vi "ModHeaderFilePar.vi"() -> ()   [LabVIEW 2019]
uses:
  Interface Class/ScanParams.ctl
  Interface Class/ScanParamsOld.ctl
  Interface Class/Interface.lvclass
panel:
  out "Header Scan":i64[](array[numeric])
  out "Session#":bool[](array[boolean])
  out "scan#":bool[](array[boolean])
  out "ScanParamsOut":T1[](array[typedef])
  out "ScanPar":i32[](array[numeric])
  out "ChainePar":string[](array[string])
  out "Session":i32[](array[numeric])
  out "Tableau 2":i32[](array[numeric])
  out "Reste session":string[](array[string])
  out "offset scan":i32[](array[numeric])
  out "ChaineSession":string[](array[string])
  out "Scan":i32[](array[numeric])
  out "Années":i32[](array[numeric])
  out "Tous Mois":i32[](array[numeric])
  out "Jours":i32[](array[numeric])
  out "ChaineReste":string[](array[string])
  out "Tableau":string[](array[string])
  out "HdrFilesNames":path[](array[path])
  in  "Data Folder Path":path
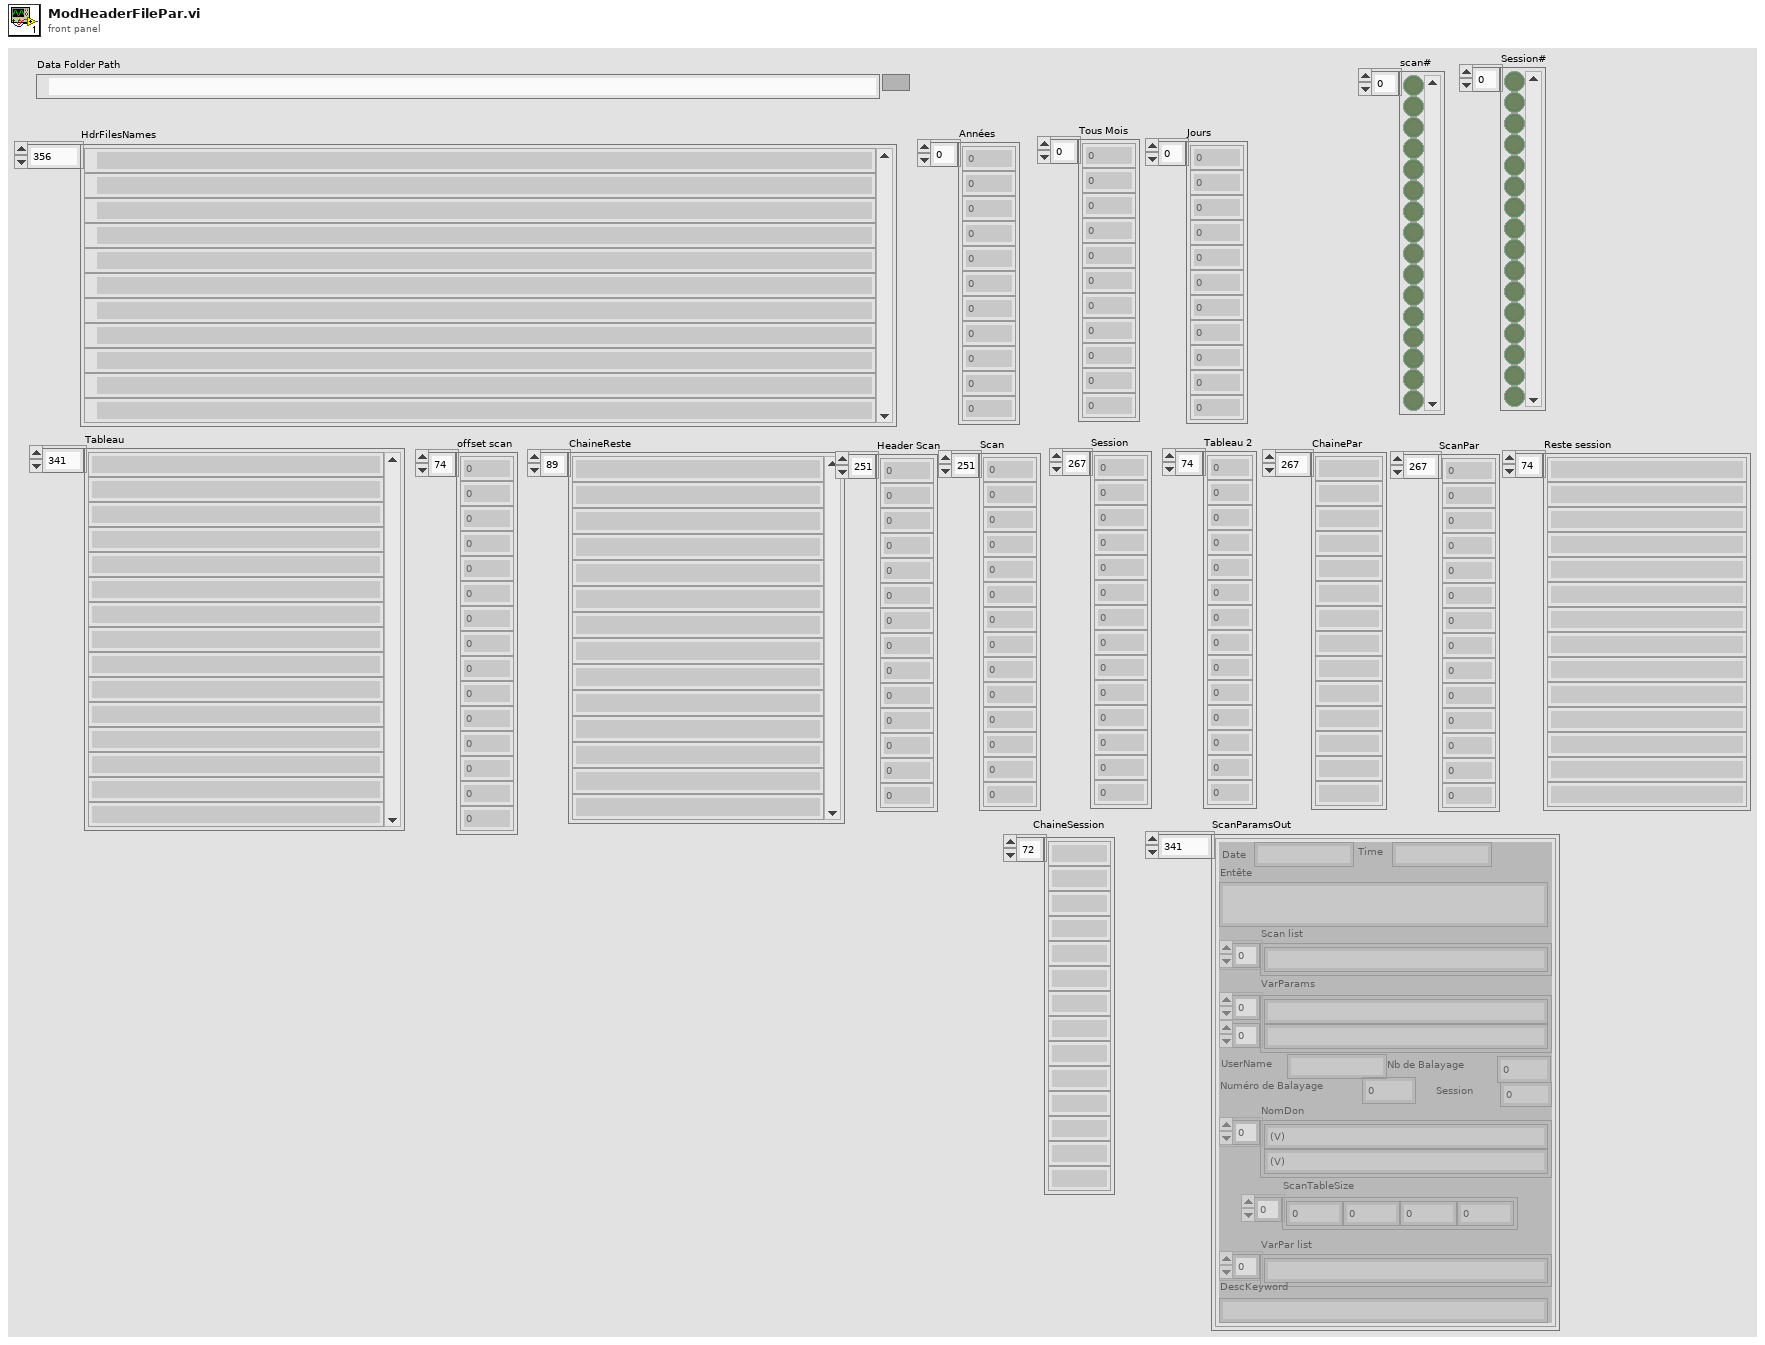
[diagram p1: front panel]
types:
  T1 = typedef "Interface.lvclass/ScanParams.ctl" = cluster{"Entête":string, "Scan list":string[], "NbCourbe":i32, "IndCourbe":i64, "NomDon":string[], "Session ":i32, "Date":string, "Time":string, "VarParams":string[][], "UserName":string, "ScanTableSize":i32[], "VarPar list":string[], "DescKeyword":string}
  T2 = typedef "Interface.lvclass/ScanParamsOld.ctl" = cluster{"Entête":string, "Scan list":string[], "NbCourbe":i32, "IndCourbe":i64, "NomDon":string[], "Session ":i32, "Date":string, "Time":string, "VarParams":string[][], "UserName":string, "ScanTableSize":i32[], "VarPar list":string[]}
  T3 = enum16{"open", "replace", "create", "open or create", "replace or create", "replace or create with confirmation"}
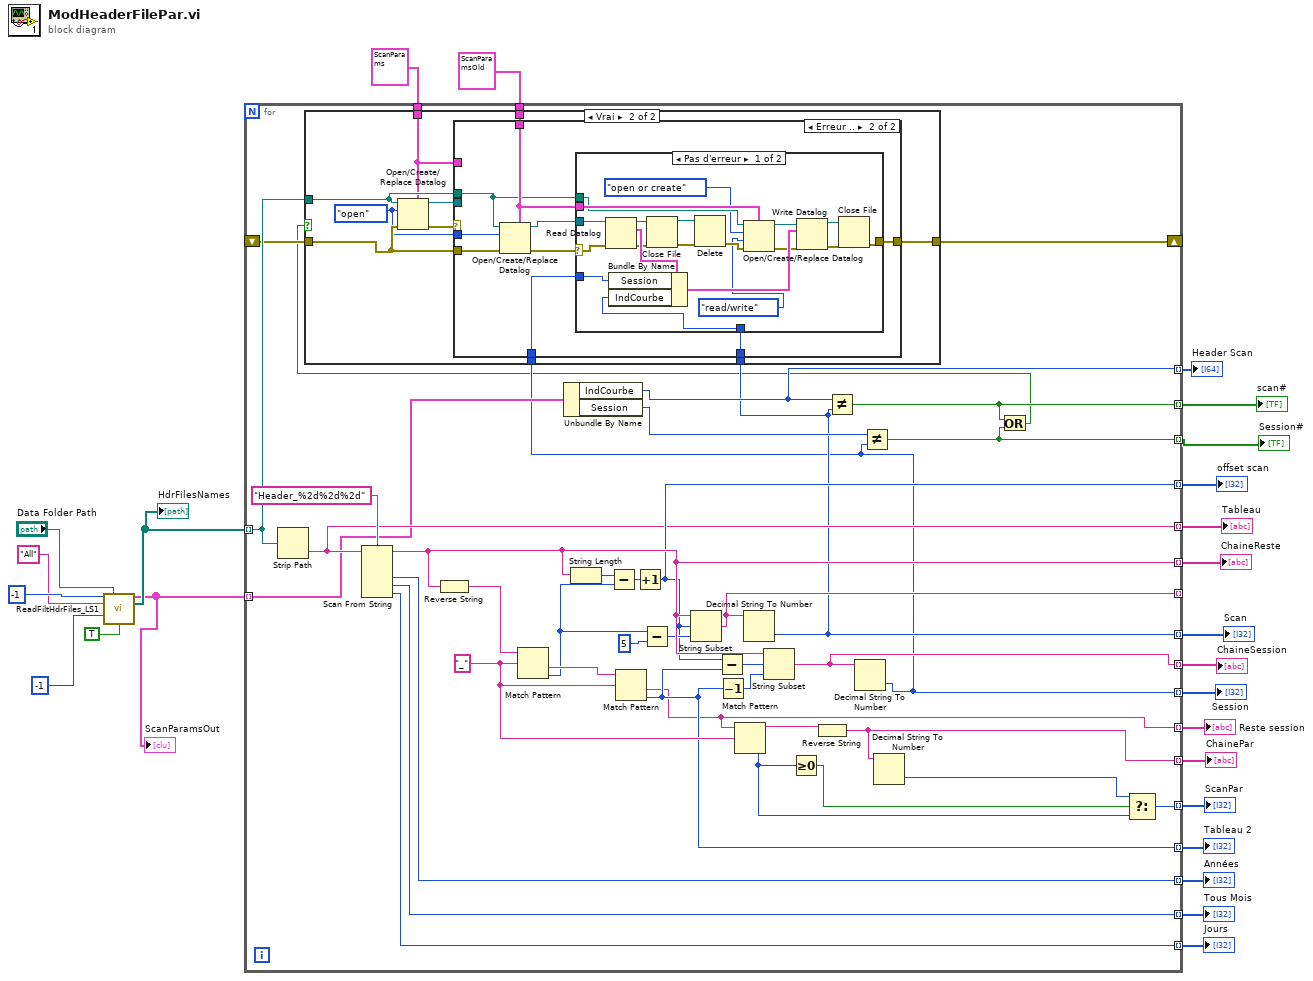
[diagram p0: block diagram]
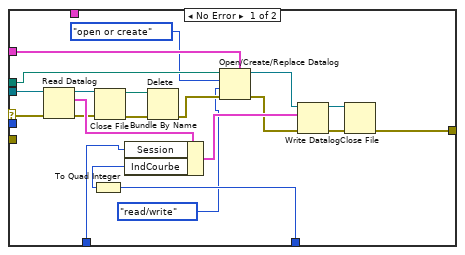
[diagram p3: hidden frame]
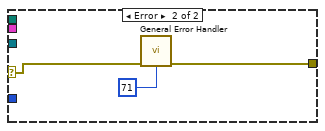
[diagram p4: hidden frame]
diagram:
  n1 = call "ReadFiltHdrFiles_LS1.vi"("nombre (-1)"=-1, "Data Folder Path"="Data Folder Path", "Date String"="All", "Session"=-1, "Recheck Files"=TRUE) -> ("ScanParamsOut"=w6:T1[], "FilesPath"=w7:path[])  [unwired: 8 in, 1 out]
  "HdrFilesNames" <- w7
  "ScanParamsOut" <- w6
  n2 = for {
    tunnel: w7 -> [w35] mode=indexing
    tunnel: [w47] -> w25 mode=indexing
    tunnel: [w58] -> w24 mode=indexing
    tunnel: [w64] -> w23 mode=indexing
    tunnel: [w63] -> w22 mode=indexing
    tunnel: [w62] -> w21 mode=indexing
    tunnel: [w30] -> w20 mode=indexing
    tunnel: [w46] -> w19 mode=indexing
    tunnel: [w56] -> _ mode=indexing
    tunnel: [w52] -> w18 mode=indexing
    tunnel: [w45] -> w17 mode=indexing
    tunnel: [w48] -> w16 mode=indexing
    tunnel: [w29] -> w15 mode=indexing
    tunnel: [w39] -> w14 mode=indexing
    tunnel: [w41] -> w13 mode=indexing
    tunnel: w6 -> [w38] mode=indexing
    tunnel: [w28] -> w5 mode=indexing
    tunnel: [w27] -> w4 mode=indexing
    tunnel: [w36] -> w3 mode=indexing
    shift-right: [w32] -> _
    shift-left: _ -> [w33]
    tunnel: T1 {"Entête"="", "Scan list"=[], "NbCourbe"=1, "IndCourbe"=1, "NomDon"=["RTêta;", "X&Y;"], "Session "=0, "Date"="", "Time"="", "VarParams"=[], "UserName"="", "ScanTableSize"=[], "VarPar list"=[], "DescKeyword"=""} ("ScanParams") -> [w34]
    tunnel: T2 {"Entête"="", "Scan list"=[], "NbCourbe"=1, "IndCourbe"=0, "NomDon"=["RTêta;", "X&Y;"], "Session "=0, "Date"="", "Time"="", "VarParams"=[], "UserName"="", "ScanTableSize"=[], "VarPar list"=[]} ("ScanParams") -> [w31]
    w60 = "_" ("expression régulière")
    n3 = Strip Path(path=w35) -> (name=w47:string)  [unwired: 1 out]
    n4 = Scan From String(format string="Header_%2d%2d%2d" ("chaîne de format"), input string=w47) -> (remaining string=w58:string, output 1=w62:i32, output 2=w63:i32, output 3=w64:i32)  [unwired: 5 in, 2 out]
    n5 = Reverse String(1:w58) -> (0:w61:string)
    n6 = Match Pattern(string=w61, regular expression=w60) -> (after substring=w51:string, offset past match=w50:i32)  [unwired: 1 in, 2 out]
    n7 = Unbundle By Name(w38) -> ("IndCourbe"=w36:i64, "Session"=w37:i32)
    n8 = String Length(string=w58) -> (length=w59:i32)
    n9 = Subtract(x=w59, y=w50) -> (x-y=w55:i32)
    n10 = Match Pattern(string=w51, regular expression=w60) -> (after substring=w45:string, offset past match=w48:i32)  [unwired: 1 in, 2 out]
    n11 = Increment(x=w55) -> (x+1=w52:i32)
    n12 = Subtract(x=w50, y=5) -> (x-y=w54:i32)
    n13 = String Subset(string=w58, offset (0)=w52, length (rest)=w54) -> (substring=w56:string)
    n14 = Subtract(x=w52, y=w48) -> (x-y=w57:i32)
    n15 = Decrement(x=w48) -> (x-1=w49:i32)
    n16 = Match Pattern(string=w45, regular expression=w60) -> (before substring=w40:string, offset past match=w42:i32)  [unwired: 1 in, 2 out]
    n17 = Decimal String To Number(string=w56) -> (number=w30:i32)  [unwired: 2 in, 1 out]
    n18 = String Subset(string=w58, offset (0)=w57, length (rest)=w49) -> (substring=w46:string)
    n19 = Greater Or Equal To 0?(x=w42) -> (x >= 0?=w43:bool)
    n20 = Reverse String(1:w40) -> (0:w39:string)
    n21 = Not Equal?(x=w36, y=w30) -> (x != y?=w28:bool)
    n22 = Decimal String To Number(string=w46) -> (number=w29:i32)  [unwired: 2 in, 1 out]
    n23 = Not Equal?(x=w37, y=w29) -> (x != y?=w27:bool)
    n24 = Decimal String To Number(string=w39) -> (number=w44:i32)  [unwired: 2 in, 1 out]
    n25 = Or(x=w28, y=w27) -> (x .or. y?=w26:bool)
    n26 = case shown="Vrai" w26 {
      tunnel: w35 -> [_ w69]
      tunnel: w34 -> [_ w67]
      tunnel: w33 -> [w66 w75]
      tunnel: [w66 w74] -> w32
      tunnel: w31 -> [_ w73]
      tunnel: w30 -> [_ w71]
      tunnel: w29 -> [_ w70]
      frame False {
      }
      frame True {
        w68 = T3."open" ("opération (0 : open)")
        n27 = Open/Create/Replace Datalog(5:w67, 8:w75, 10:w68, 11:w69) -> (0:w76:errorcluster, 3:w72:refnum<k1>)  [unwired: 2 in, 1 out]
        n28 = case shown="Erreur .." w76 {
          selector: w76 -> [w96 _]
          tunnel: w75 -> [_ w106]
          tunnel: [w90 w103] -> w74
          tunnel: w73 -> [_ w99]
          tunnel: w72 -> [w97 _]
          tunnel: w71 -> [w93 w102]
          tunnel: w70 -> [w92 w101]
          tunnel: w69 -> [w80 w98]
          tunnel: w68 -> [_ w105]
          tunnel: w67 -> [w81 _]
          frame No Error {
            n29 = Read Datalog(4:w96, 7:w97) -> (0:w87:errorcluster, 2:w95:T1, 3:w88:refnum<k1>)  [unwired: 1 in]
            n30 = To Quad Integer(1:w93) -> (0:w77:i64)
            n31 = Close File(refnum=w88, error in=w87) -> (path=w85:path, error out=w86:errorcluster)
            n32 = Bundle By Name(cluster=w95, "Session"=w92, "IndCourbe"=w77) -> (w94:T1)
            n33 = Delete(path (use dialog)=w85, error in=w86) -> (error out=w84:errorcluster)  [unwired: 3 in, 2 out]
            n34 = Open/Create/Replace Datalog(5:w81, 8:w84, 9:enum16{"read/write", "read-only", "write-only"}."read/write" ("accès (0 : read/write)"), 10:T3."open or create" ("opération (0 : open)"), 11:w80) -> (0:w83:errorcluster, 3:w82:refnum<k1>)  [unwired: 1 in, 1 out]
            n35 = Write Datalog(4:w83, 6:w94, 7:w82) -> (0:w91:errorcluster, 3:w89:refnum<k1>)
            n36 = Close File(refnum=w89, error in=w91) -> (error out=w90:errorcluster)  [unwired: 1 out]
          }
          frame Error {
            n37 = Open/Create/Replace Datalog(5:w99, 8:w106, 10:w105, 11:w98) -> (0:w104:errorcluster, 3:w100:refnum<k1>)  [unwired: 2 in, 1 out]
            n38 = case shown="Pas d'erreur" w104 {
              selector: w104 -> [w124 w128]
              tunnel: [w119 w127] -> w103
              tunnel: w102 -> [w123 _]
              tunnel: w101 -> [w122 _]
              tunnel: w100 -> [w121 _]
              tunnel: w99 -> [w112 _]
              tunnel: w98 -> [w111 _]
              frame No Error {
                n39 = Read Datalog(4:w124, 7:w121) -> (0:w116:errorcluster, 2:w126:T2, 3:w117:refnum<k1>)  [unwired: 1 in]
                n40 = Bundle By Name(cluster=w126, "Session"=w122, "IndCourbe"=w123) -> (w125:T2)
                n41 = Close File(refnum=w117, error in=w116) -> (path=w115:path, error out=w114:errorcluster)
                n42 = Delete(path (use dialog)=w115, error in=w114) -> (error out=w110:errorcluster)  [unwired: 3 in, 2 out]
                n43 = Open/Create/Replace Datalog(5:w112, 8:w110, 9:enum16{"read/write", "read-only", "write-only"}."read/write" ("accès (0 : read/write)"), 10:T3."open or create" ("opération (0 : open)"), 11:w111) -> (0:w109:errorcluster, 3:w113:refnum<k1>)  [unwired: 1 in, 1 out]
                n44 = Write Datalog(4:w109, 6:w125, 7:w113) -> (0:w120:errorcluster, 3:w118:refnum<k1>)
                n45 = Close File(refnum=w118, error in=w120) -> (error out=w119:errorcluster)  [unwired: 1 out]
              }
              frame Error {
                n46 = call <vilib>:"General Error Handler.vi"("error in (no error)"=w128, "[exception code]"=71) -> ("error out"=w127:errorcluster)  [unwired: 9 in, 4 out]
              }
            }
          }
        }
      }
    }
    n47 = Select(t=w44, s=w43, f=w42) -> (s? t:f=w41:i32)
  }
  "Tableau" <- w25
  "ChaineReste" <- w24
  "Jours" <- w23
  "Tous Mois" <- w22
  "Années" <- w21
  "Scan" <- w20
  "ChaineSession" <- w19
  "offset scan" <- w18
  "Reste session" <- w17
  "Tableau 2" <- w16
  "Session" <- w15
  "ChainePar" <- w14
  "ScanPar" <- w13
  "scan#" <- w5
  "Session#" <- w4
  "Header Scan" <- w3
